vi "1553_BC_SendMessage_Test.vi"() -> ()   [LabVIEW 2020]
uses:
  SubVIs/EXI-8000PCIe_TypeDefinitions.llb/EXI8000_MessagePrototype_Cluster.ctl
panel:
  out "Msg Returned Flag":bool
  out "StatusLoop":i32 caption="Status Loop"
  out "Msg From RT":T1={"Msg Status"=0, "Time Tag"=0, "Data.Words"=[43690, 48059, 13107, 17476, 21845, 26214], "CW"=0, "Status"=0} {"Status" format="%.0x"; "CW" format="%.0x"; "Data.Words" format="%.0x"; "Time Tag" format="%.0x"; "Msg Status" format="%.0x"}
  in  "Times to Execute Frame":i32=1
  in  "Bus":i32(ring) items=["XMT_BUS_A", "XMT_BUS_B"]
  out "Status Word\n(Hex)":i32=32768 format="%.0x"
  in  "Status.Query.Stop":bool
  in  "Min Time/Frame\n(mcrs)":i32=200 min=0
  out "Frame ID":i32
  out "Msg Id":i16=1 format="%02x"
  in  "Message Type":u16(ring)=1 format="%.0x" items=["RT2BC"=0, "BC2RT"=1, "RT2RT"=2, "MODE"=3, "BRD_RCV"=4, "BRD_RT2RT"=5, "BRD_MODE"=6, "MINOR_FRAME"=15]
  in  "Transmit/Receive":i32(ring) items=["Receive", "Transmit"]
  in  "Word Count":i32=6 min=0 max=36
  in  "RT Subaddress":i32=1 min=0 max=31
  in  "RT Num":i32=1 min=0 max=31
  in  "Data.Words":u16[](array[numeric])=[43690, 48059, 13107, 17476, 21845, 26214] format="%.0x"
  out "Mode.Get":i32(ring) format="%x" items=["RT"=2, "BC/CONCURRENT RT"=4, "MONITOR - BLOCK"=8, "MONITOR - LOOKUP"=32, "LL 0018"=68]
  out "FW Revision":i32=161
  out "Module Id":i32=69
  out "Board Status Flags":string[](array[string])=["BOARD_READY", "RAM_OK", "TIMERS_OK", "SELF_TEST_OK", "BOARD_HALTED", "PX_BOARD"]
  in  "Mode":i32(ring)=4 items=["RT"=2, "BC/CONCURRENT RT"=4, "MONITOR - BLOCK"=8, "MONITOR - LOOKUP"=32, "LL 0018"=68]
  out "Card Initialized":bool
  in  "Module":u16
  in  "Device":u16 max=255 step=1
  out "error out":errorcluster
  in  "error in":errorcluster
  # "FORMAT MESSAGE"
  # "NOTES:\n\n1. To request data from RT the\n\"Format Message\" /Transmit/Receive\nshould be set to \"Transmit\".\nThe Message Type should be set to\n\"RT2BC.\nData Words shall be empty array.\nIf the Status Word = x8201, the BC\n module did not receive data."
  # "INITIALIZE"
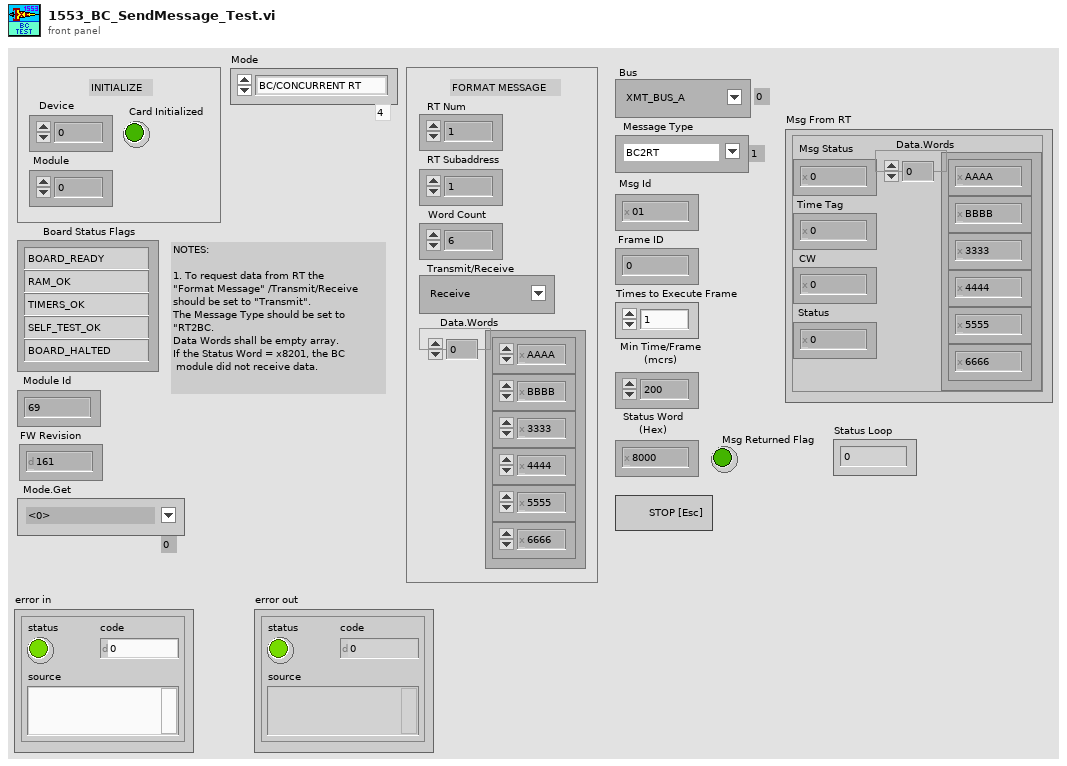
[diagram p1: front panel]
types:
  T1 = typedef "EXI8000_MessagePrototype_Cluster.ctl" = cluster{"Msg Status":u16, "Time Tag":u32, "Data.Words":u16[], "CW":u16, "Status":u16}
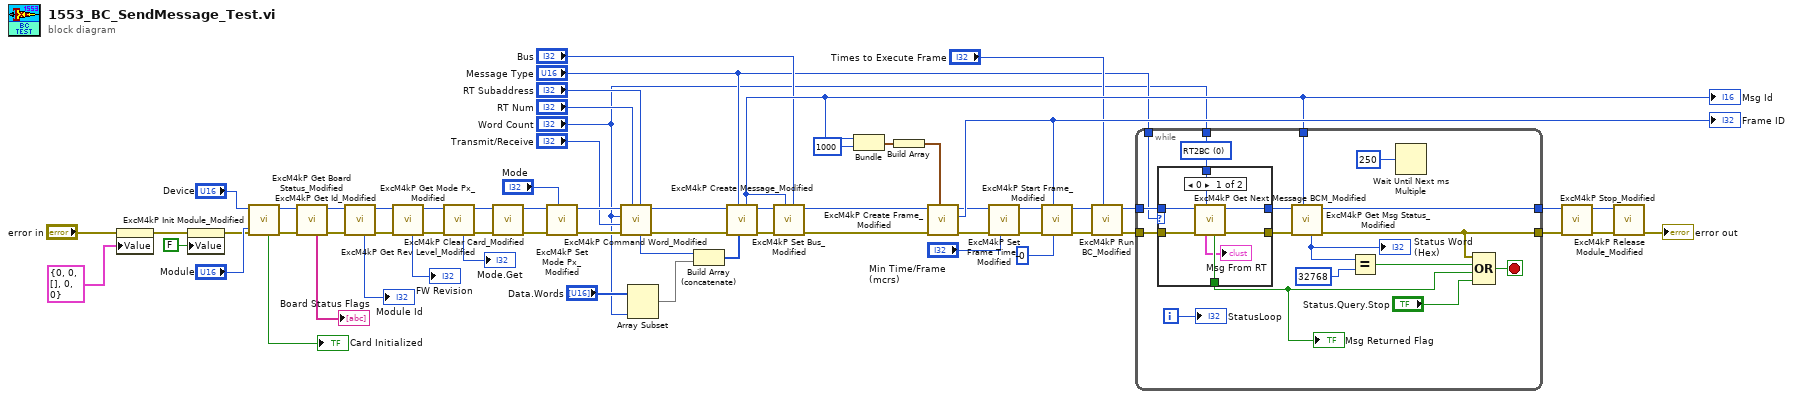
[diagram p0: block diagram]
diagram:
  n1 = property on="Msg From RT" class="Clust (strict)"(error in="error in", "Value"=T1 {"Msg Status"=0, "Time Tag"=0, "Data.Words"=[], "CW"=0, "Status"=0} ("Msg From RT")) -> (error out=w5:errorcluster)  [unwired: 1 in, 1 out]
  n2 = property on="Card Initialized" class="Bool (strict)"(error in=w5, "Value"=FALSE ("Card Initialized")) -> (error out=w60:errorcluster)  [unwired: 1 in, 1 out]
  n3 = call "ExcM4kP Init Module_Modified.vi"("Module"="Module", "error in (no error)"=w60, "Device"="Device") -> ("error out"=w51:errorcluster, "Handle"=w52:u32, "Card Initialized"=→"Card Initialized":bool)  [unwired: 6 in]
  n4 = call "ExcM4kP Get Board Status_Modified.vi"("error in (no error)"=w51, "Handle.In"=w52) -> ("error out"=w48:errorcluster, "Handle.DUP"=w49:u32, "Board Status Flags"=→"Board Status Flags":string[])  [unwired: 6 in, 1 out]
  n5 = call "ExcM4kP Get Id_Modified.vi"("error in (no error)"=w48, "Handle.In"=w49) -> ("error out"=w45:errorcluster, "Handle.DUP"=w46:u32, "Module Id"=→"Module Id":i32)  [unwired: 7 in]
  n6 = call "ExcM4kP Get Rev Level_Modified.vi"("error in (no error)"=w45, "Handle.In"=w46) -> ("error out"=w43:errorcluster, "Handle.DUP"=w42:u32, "Board.FW.Revision"=→"FW Revision":i32)  [unwired: 7 in]
  n7 = call "ExcM4kP Get Mode Px_Modified.vi"("error in (no error)"=w43, "Handle.In"=w42) -> ("error out"=w38:errorcluster, "Handle.DUP"=w40:u32, "Mode"=→"Mode.Get":i32)  [unwired: 7 in]
  n8 = call "ExcM4kP Clear Card_Modified.vi"("error in (no error)"=w38, "Handle.In"=w40) -> ("error out"=w37:errorcluster, "Handle.DUP"=w39:u32)  [unwired: 8 in]
  n9 = call "ExcM4kP Set Mode Px_Modified.vi"("Mode"="Mode", "error in (no error)"=w37, "Handle.In"=w39) -> ("error out"=w35:errorcluster, "Handle.DUP"=w36:u32)  [unwired: 7 in]
  n10 = call "ExcM4kP Command Word_Modified.vi"("RT Subaddress"="RT Subaddress", "RT Num"="RT Num", "error in (no error)"=w35, "Transmit/Receive"="Transmit/Receive", "Word Count"="Word Count", "Handle.In"=w36) -> ("error out"=w24:errorcluster, "Handle.DUP"=w23:u32, "Command Word"=w30:u16)  [unwired: 3 in]
  n11 = Array Subset(array="Data.Words", length="Word Count") -> (w29:u16[])  [unwired: 1 in]
  n12 = Build Array (concatenate)(w30, w29) -> (w28:u16[])
  n13 = call "ExcM4kP Create Message_Modified.vi"("Data"=w28, "Message Type"="Message Type", "error in (no error)"=w24, "Handle.In"=w23) -> ("error out"=w8:errorcluster, "Handle.DUP"=w9:u32, "Msg Id"=w27:i16)  [unwired: 5 in]
  "Msg Id" <- w27
  n14 = call "ExcM4kP Set Bus_Modified.vi"("Bus"="Bus", "Msg Id"=w27, "error in (no error)"=w8, "Handle.In"=w9) -> ("error out"=w3:errorcluster, "Handle.DUP"=w4:u32)  [unwired: 6 in]
  n15 = Bundle("Msg Id"=w27, 1000) -> (w21:cluster{"Msg Id":i16, i32})  [unwired: 1 out]
  n16 = Build Array(w21) -> (w20:cluster{"Msg Id":i16, i32}[])
  n17 = call "ExcM4kP Create Frame_Modified.vi"("Framestruct Array"=w20, "error in (no error)"=w3, "Handle.In"=w4) -> ("error out"=w19:errorcluster, "Frame ID"=w57:i32, "Handle.DUP"=w18:u32)  [unwired: 6 in]
  "Frame ID" <- w57
  n18 = call "ExcM4kP Set Frame Time_Modified.vi"("Min Time/Frame\n(mcrs)"="Min Time/Frame\n(mcrs)", "error in (no error)"=w19, "Handle.In"=w18) -> ("error out"=w16:errorcluster, "Handle.DUP"=w15:u32)  [unwired: 7 in]
  n19 = call "ExcM4kP Start Frame_Modified.vi"("Num Msgs to Send\n(0=All)"=0 ("Num Msgs to Send\n(0=All)"), "Frame ID"=w57, "error in (no error)"=w16, "Handle.In"=w15) -> ("error out"=w13:errorcluster, "Handle.DUP"=w12:u32)  [unwired: 6 in]
  n20 = call "ExcM4kP Run BC_Modified.vi"("Times to Execute Frame\n(0=Continuous)"="Times to Execute Frame", "error in (no error)"=w13, "Handle.In"=w12) -> ("error out"=w10:errorcluster, "Handle.DUP"=w11:u32)  [unwired: 7 in]
  n21 = while {
    tunnel: w27 -> [w80]
    tunnel: w10 -> [w70]
    tunnel: [w76] -> w53
    tunnel: w11 -> [w72]
    tunnel: [w81] -> w54
    tunnel: "Message Type" -> [w69]
    tunnel: "Word Count" -> [w66]
    i -> [w67]
    stop <- w75 stop-if-true
    (unwired) u16 0 items=["RT2BC"=0, "BC2RT"=1, "RT2RT"=2, "MODE"=3, "BRD_RCV"=4, "BRD_RT2RT"=5, "BRD_MODE"=6, "MINOR_FRAME"=15] ("Message Type")
    n22 = case shown="0" w69 {
      tunnel: [w88 w89] -> w73
      tunnel: w72 -> [w87 w89]
      tunnel: [w86 w90] -> w71
      tunnel: w70 -> [w85 w90]
      tunnel: [w84 _] -> w65
      tunnel: w66 -> [w82 _]
      frame 0 {
        n23 = call "ExcM4kP Get Next Message BCM_Modified.vi"("Word Count"=w82, "error in (no error)"=w85, "Handle.In"=w87) -> ("error out"=w86:errorcluster, "Handle.DUP"=w88:u32, "Msg Returned Flag"=w84:bool, "Msg Ptr"=→"Msg From RT":T1)  [unwired: 3 in, 2 out]
      }
      frame 1, Default {
      }
    }
    "Msg Returned Flag" <- w65
    n24 = call "ExcM4kP Get Msg Status_Modified.vi"("Msg Id"=w80, "error in (no error)"=w71, "Handle.In"=w73) -> ("error out"=w76:errorcluster, "Handle.DUP"=w81:u32, "Status Word\n(Hex)"=w78:i32)  [unwired: 6 in]
    "Status Word\n(Hex)" <- w78
    n25 = Equal?(x=w78, y=32768) -> (x = y?=w74:bool)
    n26 = Wait Until Next ms Multiple(millisecond multiple=u32 250) -> ()  [unwired: 1 out]
    n27 = Compound Arithmetic op=OR(w76, w74, w65, "Status.Query.Stop") -> (w75:bool)
    "StatusLoop" <- w67
  }
  n28 = call "ExcM4kP Stop_Modified.vi"("error in (no error)"=w53, "Handle.In"=w54) -> ("error out"=w56:errorcluster, "Handle.DUP"=w55:u32)  [unwired: 8 in]
  n29 = call "ExcM4kP Release Module_Modified.vi"("error in (no error)"=w56, "Handle.In"=w55) -> ("error out"=→"error out":errorcluster)  [unwired: 9 in]
